vi "generatepulse.vi"(6 "en":bool=TRUE, 7 "samples":i32=-1, 8 "bit":u8=1, 9 "dir":bool, 10 "kx":dbl=1.0, 11 "xn":i32=1000) -> (3 "pulsetrain":u8[](graph))   [LabVIEW 2017]
panel:
  out "Numeric":i32
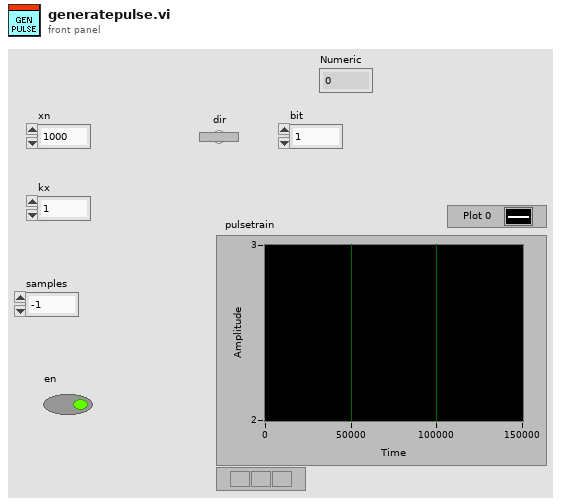
[diagram p1: front panel]
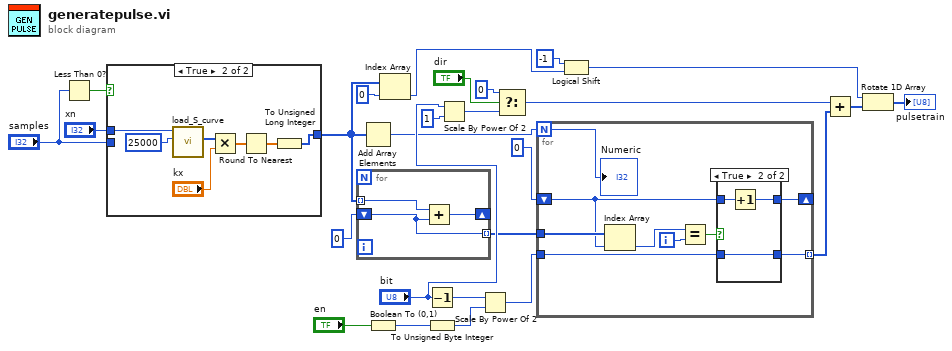
[diagram p0: block diagram]
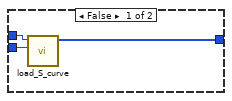
[diagram p2: hidden frame]
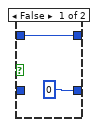
[diagram p3: hidden frame]
diagram:
  n1 = Less Than 0?(x="samples") -> (x < 0?=w14:bool)
  n2 = case shown="True" w14 {
    tunnel: "xn" -> [w29 w31]
    tunnel: [w27 w30] -> w7
    tunnel: "samples" -> [w28 _]
    frame False {
      n3 = call "load_S_curve.vi"("samples"=w28, "pulses"=w29) -> ("S Curve"=w27:u32[])  [unwired: 8 in, 1 out]
    }
    frame True {
      n4 = call "load_S_curve.vi"("samples"=25000, "pulses"=w31) -> ("Raw S Curve"=w33:u32[])  [unwired: 8 in, 1 out]
      n5 = Multiply(x=w33, y="kx") -> (x*y=w34:dbl[])
      n6 = Round To Nearest(number=w34) -> (nearest integer value=w36:dbl[])
      n7 = To Unsigned Long Integer(number=w36) -> (unsigned 32bit integer=w30:u32[])
    }
  }
  n8 = for {
    tunnel: w7 -> [w39] mode=indexing
    shift-right: [w38] -> _
    shift-left: u32 0 -> [w37]
    tunnel: [w37] -> w8 mode=indexing
    n9 = Add(x=w39, y=w37) -> (x+y=w38:u32)
  }
  n10 = Add Array Elements(numeric array=w7) -> (sum=w17:u32)
  n11 = Boolean To (0,1)(Boolean="en") -> (0, 1=w10:i16)
  n12 = Index Array(array=w7, index=0) -> (element=w5:u32)
  n13 = Decrement(x="bit") -> (x-1=w23:u8)
  n14 = To Unsigned Byte Integer(number=w10) -> (unsigned 8bit integer=w9:u8)
  n15 = Scale By Power Of 2(n="bit", x=u8 1) -> (x*2^n=w19:u8)
  n16 = Scale By Power Of 2(n=w23, x=w9) -> (x*2^n=w22:u8)
  n17 = Select(t=u8 0 ("element"), s="dir", f=w19) -> (s? t:f=w25:u8)
  n18 = for {
    N: w17 -> [w40]
    tunnel: w8 -> [w47]
    tunnel: w22 -> [w44]
    shift-right: [w41] -> _
    shift-left: u32 0 ("element") -> [w43]
    tunnel: [w42] -> w16 mode=indexing
    i -> [w48]
    n19 = Index Array(array=w47, index=w43) -> (element=w46:u32)
    n20 = Equal?(x=w46, y=w48) -> (x = y?=w45:bool)
    n21 = case shown="True" w45 {
      tunnel: w44 -> [_ w52]
      tunnel: [u8 0 ("element") w52] -> w42
      tunnel: w43 -> [w49 w53]
      tunnel: [w49 w51] -> w41
      frame False {
      }
      frame True {
        n22 = Increment(x=w53) -> (x+1=w51:u32)
      }
    }
    "Numeric" <- w40
  }
  n23 = Logical Shift(y=i16 -1, x=w5) -> (x << y=w3:u32)
  n24 = Add(x=w25, y=w16) -> (x+y=w2:u8[])
  n25 = Rotate 1D Array(1:w2, 2:w3) -> (0:→"pulsetrain":u8[])
